vi "outPutOneTestCaseInCanFile.vi"(8 "error in":errorcluster, 11 "sec+*varNoRepeatArr":string[](array[string])) -> (0 "error out":errorcluster, 3 "oneTestCaseInCanFile":string[](array[string]))   [LabVIEW 2010]
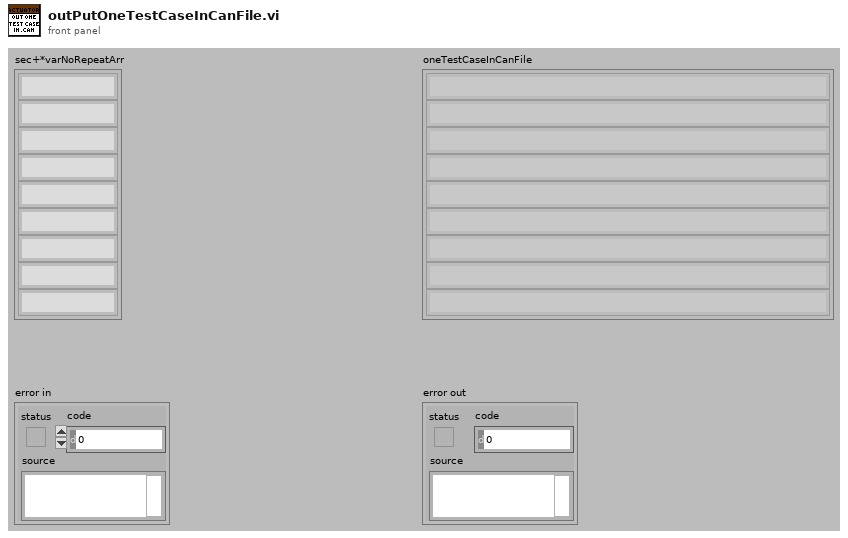
[diagram p1: front panel]
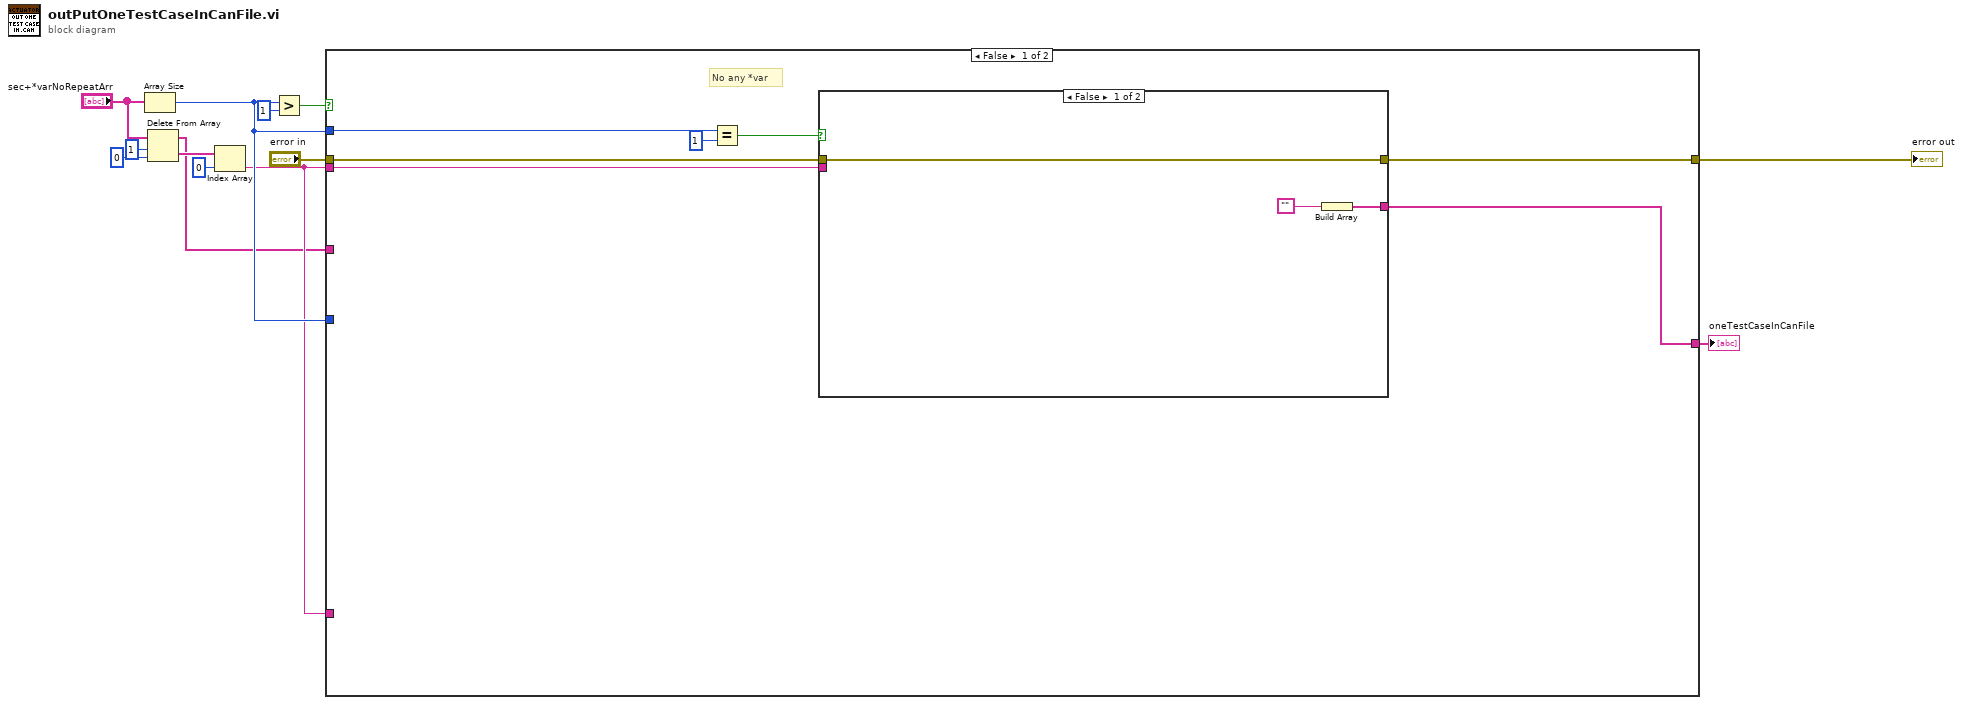
[diagram p0: block diagram]
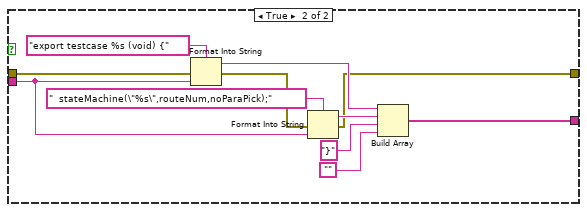
[diagram p2: hidden frame]
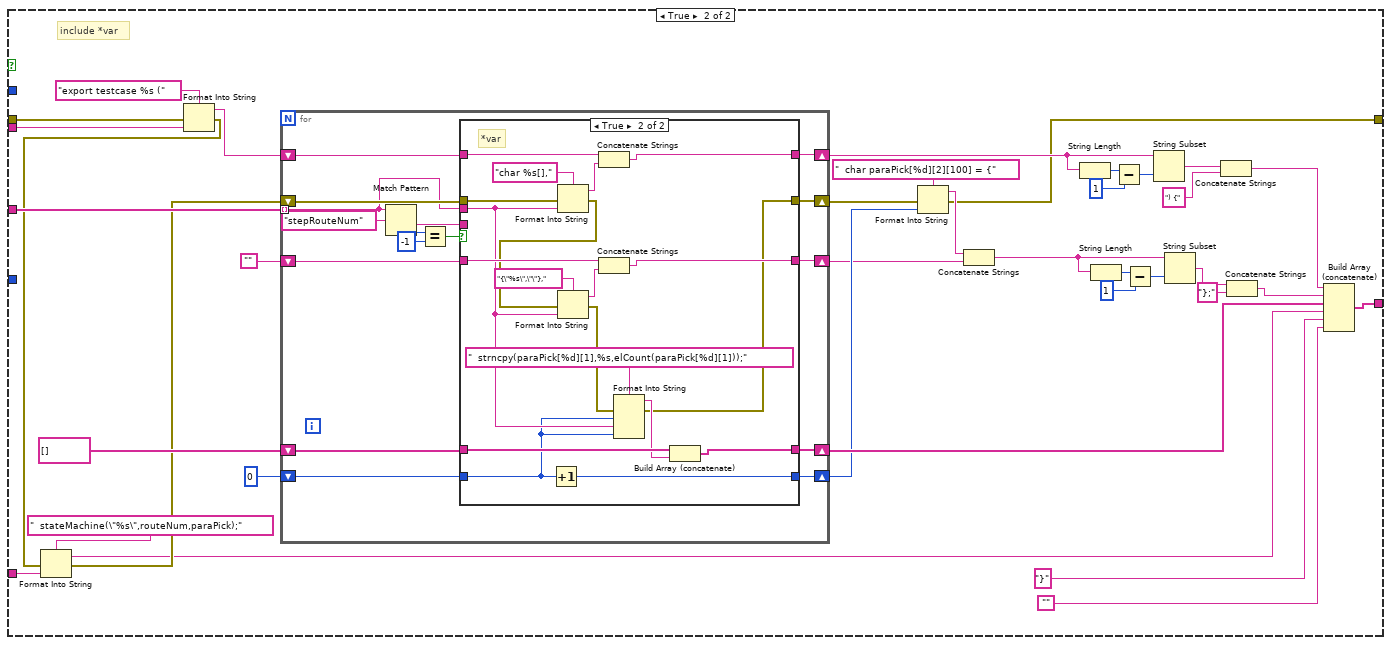
[diagram p3: hidden frame]
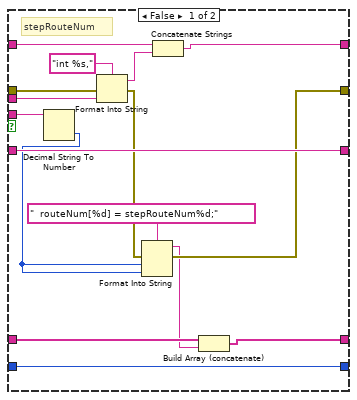
[diagram p4: hidden frame]
diagram:
  n1 = Array Size(array="sec+*varNoRepeatArr") -> (size(s)=w7:i32)
  n2 = Delete From Array(array="sec+*varNoRepeatArr", length=1, index=0) -> (deleted portion=w4:string[], array with subset deleted=w1:string[])
  n3 = Index Array(array=w4, index=0) -> (element=w2:string)
  n4 = Greater?(x=w7, y=1) -> (0:w10:bool)
  n5 = case shown="False" w10 {
    tunnel: w2 -> [w20 w45]
    tunnel: "error in" -> [w19 w70]
    tunnel: w1 -> [_ w58]
    tunnel: w7 -> [_ _]
    tunnel: w2 -> [_ w50]
    tunnel: [w18 w49] -> w12
    tunnel: [w17 w37] -> w13
    tunnel: w7 -> [w16 _]
    frame False {
      # "No any *var"
      n6 = Equal?(x=w16, y=1) -> (x = y?=w14:bool)
      n7 = case shown="False" w14 {
        tunnel: w20 -> [_ w31]
        tunnel: w19 -> [w21 w30]
        tunnel: [w22 w25] -> w18
        tunnel: [w21 w24] -> w17
        frame False {
          n8 = Build Array("") -> (w22:string[])
        }
        frame True {
          n9 = Format Into String(format string="export testcase %s (void) {", error in=w30, w31) -> (resulting string=w29:string, error out=w32:errorcluster)  [unwired: 1 in]
          n10 = Format Into String(format string="  stateMachine(\"%s\",routeNum,noParaPick);", error in=w32, w31) -> (resulting string=w28:string, error out=w24:errorcluster)  [unwired: 1 in]
          n11 = Build Array(w29, w28, "}", "") -> (w25:string[])
        }
      }
    }
    frame True {
      # "include *var"
      n12 = Format Into String(format string="export testcase %s (", error in=w70, w45) -> (resulting string=w69:string, error out=w35:errorcluster)  [unwired: 1 in]
      n13 = Format Into String(format string="  stateMachine(\"%s\",routeNum,paraPick);", error in=w35, w50) -> (resulting string=w46:string, error out=w54:errorcluster)  [unwired: 1 in]
      n14 = for {
        tunnel: w58 -> [w82] mode=indexing
        shift-right: [w74] -> w57
        shift-left: w69 -> [w84]
        shift-right: [w76] -> w38
        shift-left: "" -> [w81]
        shift-right: [w73] -> w51
        shift-left: string[] [] -> [w80]
        shift-right: [w75] -> w41
        shift-left: w54 -> [w83]
        shift-right: [w77] -> w40
        shift-left: 0 ("index") -> [w78]
        n15 = Match Pattern(string=w82, regular expression="stepRouteNum" ("format string")) -> (after substring=w72:string, offset past match=w86:i32)  [unwired: 1 in, 2 out]
        n16 = Equal?(x=w86, y=-1) -> (x = y?=w79:bool)
        n17 = case shown="True" w79 {
          tunnel: w84 -> [w103 w122]
          tunnel: [w96 w121] -> w76
          tunnel: [w98 w116] -> w74
          tunnel: w81 -> [w96 w115]
          tunnel: w82 -> [w100 w113]
          tunnel: w80 -> [w90 w112]
          tunnel: [w88 w110] -> w73
          tunnel: w83 -> [w101 w109]
          tunnel: [w91 w106] -> w75
          tunnel: w78 -> [w97 w104]
          tunnel: [w97 w105] -> w77
          tunnel: w72 -> [w95 _]
          frame False {
            # "stepRouteNum"
            n18 = Decimal String To Number(string=w95) -> (number=w93:i32)  [unwired: 2 in, 1 out]
            n19 = Format Into String(format string="int %s,", error in=w101, w100) -> (resulting string=w99:string, error out=w92:errorcluster)  [unwired: 1 in]
            n20 = Format Into String(format string="  routeNum[%d] = stepRouteNum%d;", error in=w92, w93, w93) -> (resulting string=w89:string, error out=w91:errorcluster)  [unwired: 1 in]
            n21 = Concatenate Strings(w103, w99) -> (w98:string)
            n22 = Build Array (concatenate)(w90, w89) -> (w88:string[])
          }
          frame True {
            # "*var"
            n23 = Increment(x=w104) -> (x+1=w105:i32)
            n24 = Format Into String(format string="char %s[],", error in=w109, w113) -> (resulting string=w117:string, error out=w108:errorcluster)  [unwired: 1 in]
            n25 = Format Into String(format string="{\"%s\",\"\"},", error in=w108, w113) -> (resulting string=w119:string, error out=w107:errorcluster)  [unwired: 1 in]
            n26 = Concatenate Strings(w122, w117) -> (w116:string)
            n27 = Concatenate Strings(w115, w119) -> (w121:string)
            n28 = Format Into String(format string="  strncpy(paraPick[%d][1],%s,elCount(paraPick[%d][1]));", error in=w107, w104, w113, w104) -> (resulting string=w111:string, error out=w106:errorcluster)  [unwired: 1 in]
            n29 = Build Array (concatenate)(w112, w111) -> (w110:string[])
          }
        }
      }
      n30 = Format Into String(format string="  char paraPick[%d][2][100] = {", error in=w41, w40) -> (resulting string=w39:string, error out=w37:errorcluster)  [unwired: 1 in]
      n31 = Concatenate Strings(w39, w38) -> (w36:string)
      n32 = String Length(string=w57) -> (length=w64:i32)
      n33 = String Length(string=w36) -> (length=w63:i32)
      n34 = Subtract(x=w64, y=1) -> (x-y=w66:i32)
      n35 = Subtract(x=w63, y=1) -> (x-y=w61:i32)
      n36 = String Subset(string=w57, length (rest)=w66) -> (substring=w67:string)  [unwired: 1 in]
      n37 = String Subset(string=w36, length (rest)=w61) -> (substring=w60:string)  [unwired: 1 in]
      n38 = Concatenate Strings(w67, ") {" ("sec")) -> (w53:string)
      n39 = Concatenate Strings(w60, "};" ("string")) -> (w52:string)
      n40 = Build Array (concatenate)(w53, w52, w51, w46, "}" ("string"), "") -> (w49:string[])
    }
  }
  "error out" <- w13
  "oneTestCaseInCanFile" <- w12
